vi "Activate Menu Items.vi"(8 "error in (no error)":errorcluster, 9 "State(0)":i32, 10 "MenuRefnum":refnum<k9>, 11 "Menu in":refnum<class "Menu.lvclass">) -> (0 "error out":errorcluster, 3 "Menu out":refnum<class "Menu.lvclass">)   [LabVIEW 2015, in "Menu.lvclass"]
uses:
  Menu.lvclass
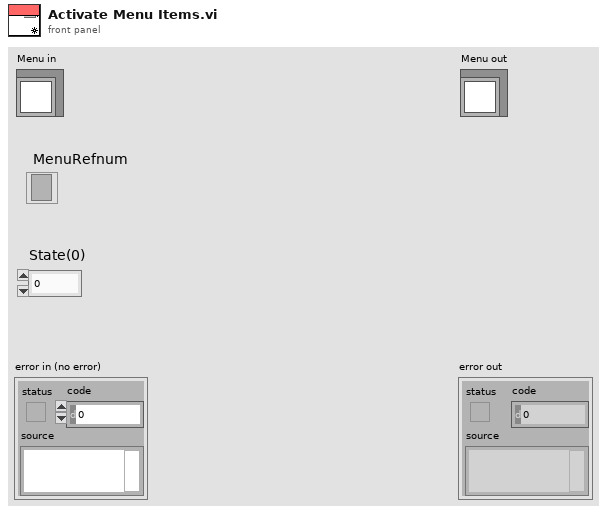
[diagram p1: front panel]
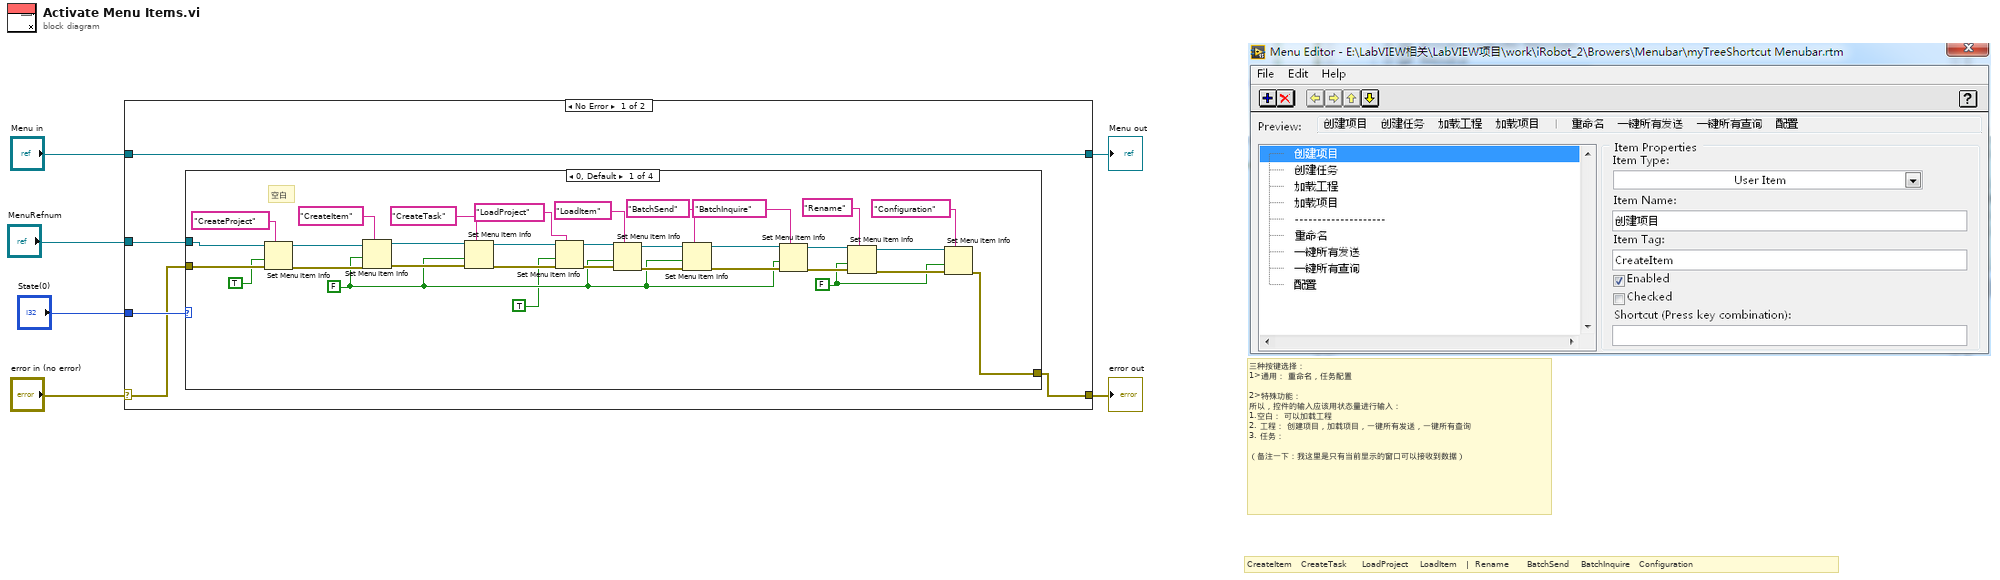
[diagram p0: block diagram]
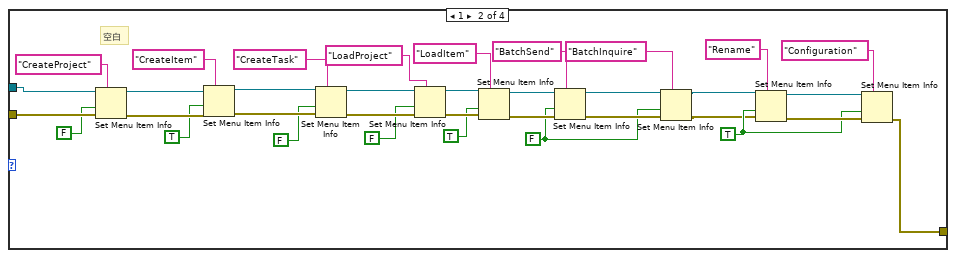
[diagram p2: hidden frame]
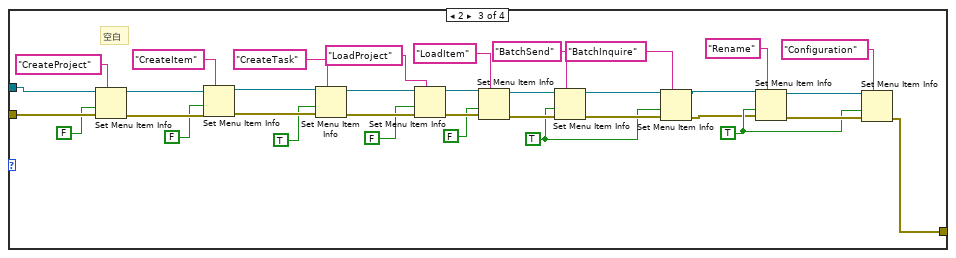
[diagram p3: hidden frame]
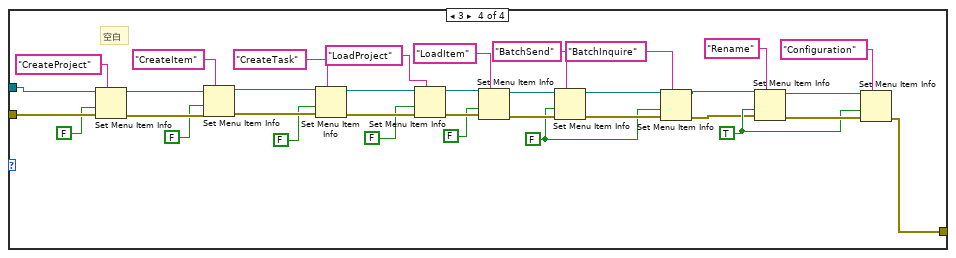
[diagram p4: hidden frame]
diagram:
  # "CreateItem   CreateTask     LoadProject    LoadItem   |  Rename      BatchSend    BatchInquire   Configuration"
  # "三种按键选择：\n1>通用： 重命名，任务配置\n\n2>特殊功能：\n所以，控件的输入应该用状态量进行输入：\n1.空白： 可以加载工程\n2. 工程： 创建项目，加载项目，一键所有发送，一键所有查询\n3. 任务：\n\n（备注一下：我这里是只有当前显示的窗口可以接收到数据）"
  n1 = case shown="No Error" "error in (no error)" {
    selector: "error in (no error)" -> [w8 w150]
    tunnel: [w7 w150] -> w5
    tunnel: [w11 w149] -> w3
    tunnel: "Menu in" -> [w11 w149]
    tunnel: "MenuRefnum" -> [w10 _]
    tunnel: "State(0)" -> [w9 _]
    frame No Error {
      n2 = case shown="0, Default" w9 {
        tunnel: w10 -> [w27 w62 w97 w132]
        tunnel: w8 -> [w26 w61 w96 w131]
        tunnel: [w13 w44 w79 w114] -> w7
        frame 0, Default {
          w12 = FALSE ("enabled")
          w23 = FALSE ("enabled")
          # "空白"
          n3 = Set Menu Item Info(7:"CreateProject" ("item tag"), 8:w26, 9:TRUE ("enabled"), 11:w27) -> (0:w29:errorcluster, 3:w28:refnum<k9>)  [unwired: 3 in]
          n4 = Set Menu Item Info(7:"CreateItem" ("item tag"), 8:w29, 9:w23, 11:w28) -> (0:w40:errorcluster, 3:w41:refnum<k9>)  [unwired: 3 in]
          n5 = Set Menu Item Info(7:"CreateTask" ("item tag"), 8:w40, 9:w23, 11:w41) -> (0:w38:errorcluster, 3:w39:refnum<k9>)  [unwired: 3 in]
          n6 = Set Menu Item Info(7:"LoadProject" ("item tag"), 8:w38, 9:TRUE ("enabled"), 11:w39) -> (0:w36:errorcluster, 3:w37:refnum<k9>)  [unwired: 3 in]
          n7 = Set Menu Item Info(7:"LoadItem" ("item tag"), 8:w36, 9:w23, 11:w37) -> (0:w33:errorcluster, 3:w34:refnum<k9>)  [unwired: 3 in]
          n8 = Set Menu Item Info(7:"BatchSend" ("item tag"), 8:w33, 9:w23, 11:w34) -> (0:w31:errorcluster, 3:w30:refnum<k9>)  [unwired: 3 in]
          n9 = Set Menu Item Info(7:"BatchInquire" ("item tag"), 8:w31, 9:w23, 11:w30) -> (0:w18:errorcluster, 3:w19:refnum<k9>)  [unwired: 3 in]
          n10 = Set Menu Item Info(7:"Rename" ("item tag"), 8:w18, 9:w12, 11:w19) -> (0:w15:errorcluster, 3:w16:refnum<k9>)  [unwired: 3 in]
          n11 = Set Menu Item Info(7:"Configuration" ("item tag"), 8:w15, 9:w12, 11:w16) -> (0:w13:errorcluster)  [unwired: 3 in, 1 out]
        }
        frame 1 {
          w47 = TRUE ("enabled")
          w54 = FALSE ("enabled")
          # "空白"
          n12 = Set Menu Item Info(7:"CreateProject" ("item tag"), 8:w61, 9:FALSE ("enabled"), 11:w62) -> (0:w64:errorcluster, 3:w63:refnum<k9>)  [unwired: 3 in]
          n13 = Set Menu Item Info(7:"CreateItem" ("item tag"), 8:w64, 9:TRUE ("enabled"), 11:w63) -> (0:w75:errorcluster, 3:w76:refnum<k9>)  [unwired: 3 in]
          n14 = Set Menu Item Info(7:"CreateTask" ("item tag"), 8:w75, 9:FALSE ("enabled"), 11:w76) -> (0:w73:errorcluster, 3:w74:refnum<k9>)  [unwired: 3 in]
          n15 = Set Menu Item Info(7:"LoadProject" ("item tag"), 8:w73, 9:FALSE ("enabled"), 11:w74) -> (0:w71:errorcluster, 3:w72:refnum<k9>)  [unwired: 3 in]
          n16 = Set Menu Item Info(7:"LoadItem" ("item tag"), 8:w71, 9:TRUE ("enabled"), 11:w72) -> (0:w68:errorcluster, 3:w69:refnum<k9>)  [unwired: 3 in]
          n17 = Set Menu Item Info(7:"BatchSend" ("item tag"), 8:w68, 9:w54, 11:w69) -> (0:w66:errorcluster, 3:w65:refnum<k9>)  [unwired: 3 in]
          n18 = Set Menu Item Info(7:"BatchInquire" ("item tag"), 8:w66, 9:w54, 11:w65) -> (0:w45:errorcluster, 3:w46:refnum<k9>)  [unwired: 3 in]
          n19 = Set Menu Item Info(7:"Rename" ("item tag"), 8:w45, 9:w47, 11:w46) -> (0:w49:errorcluster, 3:w50:refnum<k9>)  [unwired: 3 in]
          n20 = Set Menu Item Info(7:"Configuration" ("item tag"), 8:w49, 9:w47, 11:w50) -> (0:w44:errorcluster)  [unwired: 3 in, 1 out]
        }
        frame 2 {
          w82 = TRUE ("enabled")
          w89 = TRUE ("enabled")
          # "空白"
          n21 = Set Menu Item Info(7:"CreateProject" ("item tag"), 8:w96, 9:FALSE ("enabled"), 11:w97) -> (0:w99:errorcluster, 3:w98:refnum<k9>)  [unwired: 3 in]
          n22 = Set Menu Item Info(7:"CreateItem" ("item tag"), 8:w99, 9:FALSE ("enabled"), 11:w98) -> (0:w110:errorcluster, 3:w111:refnum<k9>)  [unwired: 3 in]
          n23 = Set Menu Item Info(7:"CreateTask" ("item tag"), 8:w110, 9:TRUE ("enabled"), 11:w111) -> (0:w108:errorcluster, 3:w109:refnum<k9>)  [unwired: 3 in]
          n24 = Set Menu Item Info(7:"LoadProject" ("item tag"), 8:w108, 9:FALSE ("enabled"), 11:w109) -> (0:w106:errorcluster, 3:w107:refnum<k9>)  [unwired: 3 in]
          n25 = Set Menu Item Info(7:"LoadItem" ("item tag"), 8:w106, 9:FALSE ("enabled"), 11:w107) -> (0:w103:errorcluster, 3:w104:refnum<k9>)  [unwired: 3 in]
          n26 = Set Menu Item Info(7:"BatchSend" ("item tag"), 8:w103, 9:w89, 11:w104) -> (0:w101:errorcluster, 3:w100:refnum<k9>)  [unwired: 3 in]
          n27 = Set Menu Item Info(7:"BatchInquire" ("item tag"), 8:w101, 9:w89, 11:w100) -> (0:w80:errorcluster, 3:w81:refnum<k9>)  [unwired: 3 in]
          n28 = Set Menu Item Info(7:"Rename" ("item tag"), 8:w80, 9:w82, 11:w81) -> (0:w84:errorcluster, 3:w85:refnum<k9>)  [unwired: 3 in]
          n29 = Set Menu Item Info(7:"Configuration" ("item tag"), 8:w84, 9:w82, 11:w85) -> (0:w79:errorcluster)  [unwired: 3 in, 1 out]
        }
        frame 3 {
          w117 = TRUE ("enabled")
          w124 = FALSE ("enabled")
          # "空白"
          n30 = Set Menu Item Info(7:"CreateProject" ("item tag"), 8:w131, 9:FALSE ("enabled"), 11:w132) -> (0:w134:errorcluster, 3:w133:refnum<k9>)  [unwired: 3 in]
          n31 = Set Menu Item Info(7:"CreateItem" ("item tag"), 8:w134, 9:FALSE ("enabled"), 11:w133) -> (0:w145:errorcluster, 3:w146:refnum<k9>)  [unwired: 3 in]
          n32 = Set Menu Item Info(7:"CreateTask" ("item tag"), 8:w145, 9:FALSE ("enabled"), 11:w146) -> (0:w143:errorcluster, 3:w144:refnum<k9>)  [unwired: 3 in]
          n33 = Set Menu Item Info(7:"LoadProject" ("item tag"), 8:w143, 9:FALSE ("enabled"), 11:w144) -> (0:w141:errorcluster, 3:w142:refnum<k9>)  [unwired: 3 in]
          n34 = Set Menu Item Info(7:"LoadItem" ("item tag"), 8:w141, 9:FALSE ("enabled"), 11:w142) -> (0:w138:errorcluster, 3:w139:refnum<k9>)  [unwired: 3 in]
          n35 = Set Menu Item Info(7:"BatchSend" ("item tag"), 8:w138, 9:w124, 11:w139) -> (0:w136:errorcluster, 3:w135:refnum<k9>)  [unwired: 3 in]
          n36 = Set Menu Item Info(7:"BatchInquire" ("item tag"), 8:w136, 9:w124, 11:w135) -> (0:w115:errorcluster, 3:w116:refnum<k9>)  [unwired: 3 in]
          n37 = Set Menu Item Info(7:"Rename" ("item tag"), 8:w115, 9:w117, 11:w116) -> (0:w119:errorcluster, 3:w120:refnum<k9>)  [unwired: 3 in]
          n38 = Set Menu Item Info(7:"Configuration" ("item tag"), 8:w119, 9:w117, 11:w120) -> (0:w114:errorcluster)  [unwired: 3 in, 1 out]
        }
      }
    }
    frame Error {
    }
  }
  "error out" <- w5
  "Menu out" <- w3
